vi "pop.vi"() -> (0 "Data out":dbl[][](array[numeric]))   [LabVIEW 2013]
uses:
  GlobleVar/Data.vi
  GlobleVar/ptr_write.vi
  GlobleVar/segment_size.vi
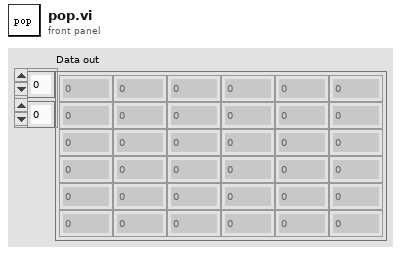
[diagram p1: front panel]
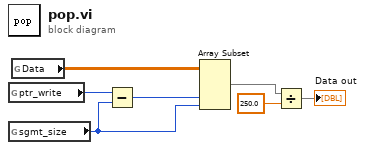
[diagram p0: block diagram]
diagram:
  n1 = global read "ptr_write.vi" "ptr_write"() -> (w5:i32)
  n2 = global read "segment_size.vi" "sgmt_size"() -> (w6:i32)
  n3 = global read "Data.vi" "Data"() -> (w7:dbl[][])
  n4 = Subtract(x=w5, y=w6) -> (x-y=w4:i32)
  n5 = Array Subset(array=w7, index (col)=w4, length (col)=w6) -> (w1:dbl[][])  [unwired: 2 in]
  n6 = Divide(x=w1, y=250.0) -> (x/y=→"Data out":dbl[][])
